vi "Extract Diagram Text.vi"(8 "error in (no error)":errorcluster, 9 "Label Prefix":string, 10 "DiagObjRefs[]":refnum<vi>[](array[refnum]), 11 "VI Data in":refnum<class "VI Data.lvclass">) -> (0 "error out":errorcluster, 3 "VI Data out":refnum<class "VI Data.lvclass">)   [LabVIEW 2013, in "SET Project Data.lvlib" / "VI Data.lvclass"]
uses:
  VI Data.lvclass
  VI Data.lvclass/VI Data.ctl
  Control Classes/GObject/GObject.lvclass
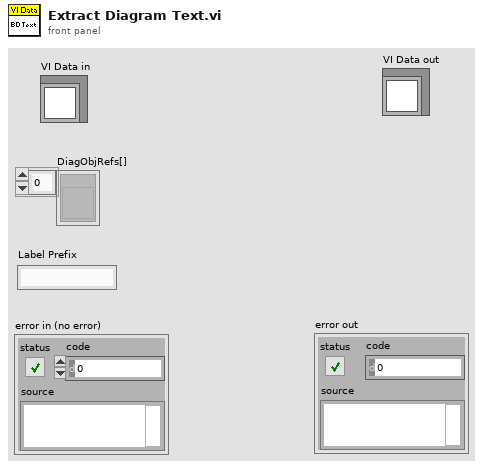
[diagram p1: front panel]
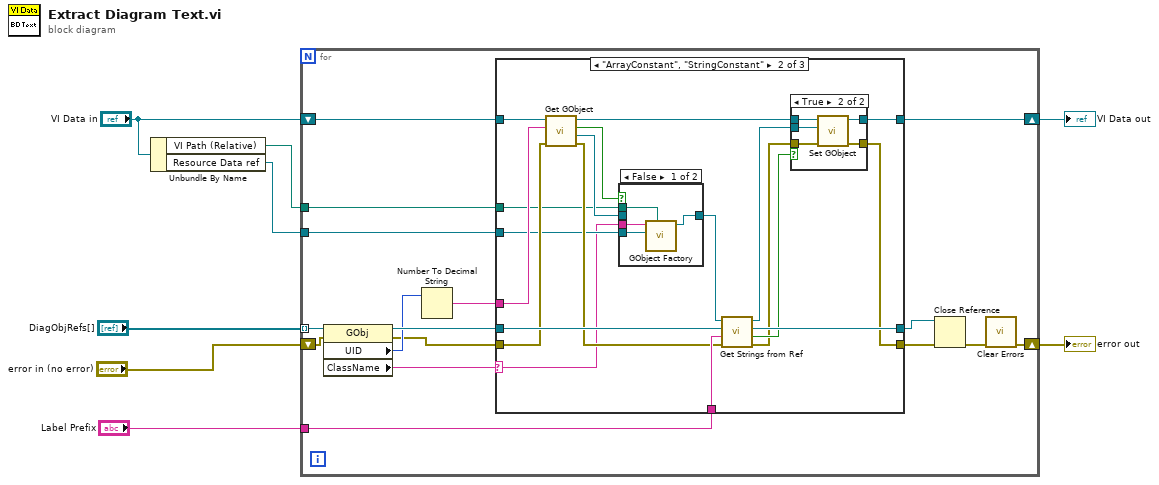
[diagram p0: block diagram]
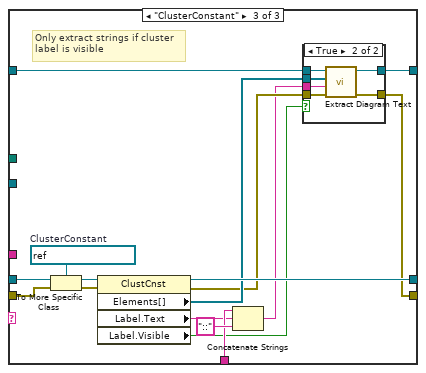
[diagram p5: hidden frame]
diagram:
  n1 = Unbundle By Name("VI Data in") -> ("VI Path (Relative)"=w4:path, "Resource Data ref"=w3:refnum<data-value>)
  n2 = for {
    tunnel: "DiagObjRefs[]" -> [w20] mode=indexing
    shift-right: [w23] -> w6
    shift-left: "error in (no error)" -> [w19]
    tunnel: "Label Prefix" -> [w22]
    tunnel: w3 -> [w12]
    tunnel: w4 -> [w13]
    shift-right: [w9] -> w1
    shift-left: "VI Data in" -> [w14]
    n3 = property class="GObj"(reference=w20, error in=w19) -> (reference out=w18:refnum<vi>, error out=w15:errorcluster, "UID"=w17:i32, "ClassName"=w11:string)
    n4 = Number To Decimal String(number=w17) -> (decimal integer string=w16:string)  [unwired: 1 in]
    n5 = case shown="\"ArrayConstant\", \"StringConstant\"" w11 {
      selector: w11 -> [_ w28 _]
      tunnel: w18 -> [w27 w44 w74]
      tunnel: [w27 w45 w69] -> w21
      tunnel: w15 -> [w26 w39 w73]
      tunnel: [w26 w29 w66] -> w10
      tunnel: w22 -> [_ w46 w63]
      tunnel: w16 -> [_ w41 _]
      tunnel: w14 -> [w25 w40 w60]
      tunnel: [w25 w33 w59] -> w9
      tunnel: w13 -> [_ w37 _]
      tunnel: w12 -> [_ w36 _]
      frame Default {
      }
      frame "ArrayConstant", "StringConstant" {
        n6 = call-dynamic "Get GObject.vi"("error in (no error)"=w39, "GObject UID"=w41, "VI Data in"=w40) -> ("error out"=w38:errorcluster, "GObject"=w43:refnum<class "GObject.lvclass">, "found"=w42:bool, "VI Data out"=w34:refnum<class "VI Data.lvclass">)  [unwired: 5 in]
        n7 = case shown="False" w42 {
          tunnel: w28 -> [w57 _]
          tunnel: w36 -> [w56 _]
          tunnel: w37 -> [w55 _]
          tunnel: w43 -> [_ w58]
          tunnel: [w54 w58] -> w35
          frame False {
            n8 = call "GObject Factory.vi"("Owning VI"=w55, "LangFile ref"=w56, "ClassName"=w57) -> ("GObject"=w54:refnum<class "GObject.lvclass">)  [unwired: 8 in]
          }
          frame True {
          }
        }
        n9 = call-dynamic "Get Strings from Ref.vi"("error in (no error)"=w38, "Label Prefix"=w46, "GObj Refnum in"=w44, "GObject in"=w35) -> ("error out"=w30:errorcluster, "Valid?"=w31:bool, "GObj Refnum out"=w45:refnum<vi>, "GObject out"=w32:refnum<class "GObject.lvclass">)  [unwired: 3 in, 1 out]
        n10 = case shown="True" w31 {
          tunnel: w34 -> [w48 w53]
          tunnel: [w48 w52] -> w33
          tunnel: w32 -> [_ w51]
          tunnel: w30 -> [w47 w50]
          tunnel: [w47 w49] -> w29
          frame False {
          }
          frame True {
            n11 = call "Set GObject.vi"("error in (no error)"=w50, "GObject.lvclass"=w51, "VI Data in"=w53) -> ("error out"=w49:errorcluster, "VI Data out"=w52:refnum<class "VI Data.lvclass">)  [unwired: 6 in, 1 out]
          }
        }
      }
      frame "ClusterConstant" {
        w72 = refnum<vi> refnum  # ClusterConstant
        # "Only extract strings if cluster\nlabel is visible"
        n12 = To More Specific Class(target class=w72, reference=w74, error in=w73) -> (specific class reference=w71:refnum<vi>, error out=w70:errorcluster)
        n13 = property class="ClustCnst"(reference=w71, error in=w70) -> (reference out=w69:refnum<vi>, error out=w67:errorcluster, "Elements[]"=w68:refnum<vi>[], "Label.Text"=w62:string, "Label.Visible"=w61:bool)
        n14 = Concatenate Strings(w63, w62, "::" ("string")) -> (w64:string)
        n15 = case shown="True" w61 {
          tunnel: w60 -> [w76 w82]
          tunnel: [w76 w81] -> w59
          tunnel: w68 -> [_ w80]
          tunnel: w67 -> [w75 w79]
          tunnel: [w75 w78] -> w66
          tunnel: w64 -> [_ w77]
          frame False {
          }
          frame True {
            n16 = call "Extract Diagram Text.vi"("error in (no error)"=w79, "Label Prefix"=w77, "DiagObjRefs[]"=w80, "VI Data in"=w82) -> ("error out"=w78:errorcluster, "VI Data out"=w81:refnum<class "VI Data.lvclass">)  [unwired: 6 in]
          }
        }
      }
    }
    n17 = Close Reference(reference=w21, error in (no error)=w10) -> (error out=w24:errorcluster)
    n18 = call <vilib>:"Clear Errors.vi"("error in (no error)"=w24) -> ("error out"=w23:errorcluster)  [unwired: 6 in]
  }
  "error out" <- w6
  "VI Data out" <- w1
